vi "Runtime.vi"() -> ()   [LabVIEW 2025]
uses:
  <vilib>/Platform/TimedLoop/XDataNode/timing_clust.ctl
  <vilib>/Platform/TimedLoop/XDataNode/nitl_modes.ctl
  <vilib>/Platform/TimedLoop/XDataNode/wakeup.ctl
  <vilib>/Analysis/5stat.llb/RMS (DBL).vi
  <vilib>/platform/TimedLoop/XDataNode/XDataNode.xnode
  <vilib>/Platform/TimedLoop/XDataNode/XDNodeRunTimeDep.lvlib
  <vilib>/Analysis/NI_AALBase.lvlib
  <vilib>/ptbypt/NI_PtbyPt.lvlib
  <vilib>/Analysis/NI_AALPro.lvlib
panel:
  in  "結束":bool
  out "Velocity":dbl[](graph)
  out "Initial position":i32
  in  "產生路徑":bool
  out "after servo on":u16 format="%.0b"
  out "Initial target velocity":i32
  out "statusword":u16 format="%.0b"
  out "1st Transmit PDO Mapping-Modes of operation display":i8
  in  "Servo on":bool
  in  "1st Receive PDO Mapping-Controlword":u16=128 format="%.0b"
  in  "Fault reset":bool
  in  "STOP":bool
  out "rms error":dbl format="%0.2f"
  out "TCP":errorcluster
  out "Error":string
  out "Done 2":bool caption="TCP Done"
  out "Path":dbl[](graph)
  out "Output":dbl[](graph)
  out "Error":dbl[](graph)
  out "限制上限":bool
  out "Delay":i32
  out "Done":bool caption="Run Done"
  in  "停止":bool
  in  "開始執行":bool
  out "data length":i32
  out "pdl":i32
  out "Total time":i32
  out "Ts":dbl=0.001
  # "資料儲存區"
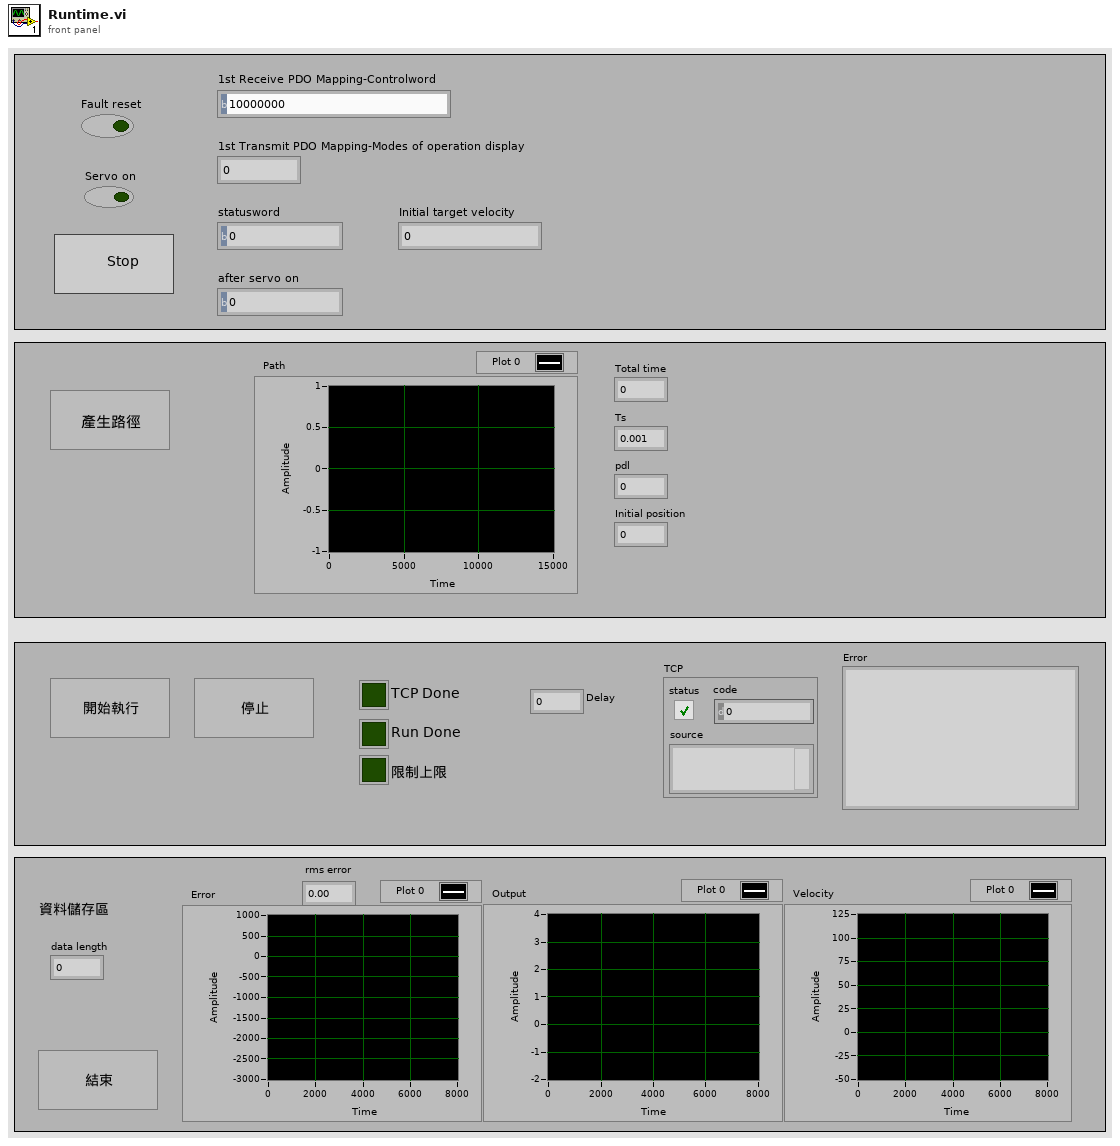
[diagram p1: front panel]
types:
  T1 = typedef "XDNodeRunTimeDep.lvlib/timing_clust.ctl" = cluster{"Expected End [f-1]":u64, "Actual End [f-1]":u64, "Finished Late? [f-1]":bool, "Expected End [i-1]":u64, "Actual End [i-1]":u64, "Finished Late? [i-1]":bool, "Expected Start [i]":u64, "Actual Start [i]":u64, "Expected Start [f]":u64, "Actual Start [f]":u64, "Source Name":string, "Structure Name":string, "Period":i64, "Deadline":i64, "Offset":i64, "Start":i64, "Priority":i32, "Timeout":i32, "Mode":T2, "Wakeup Reason":T3, "Error":errorcluster, "Source Type":string, "Secondary Source Type":string, "Global End Time":u64, "Global Start Time":u64, "Frame Duration":u64, "Iteration Duration":u64, "Assigned CPU":i32, "I/O Scan Engine Mode":u32}
  T2 = typedef "XDNodeRunTimeDep.lvlib/nitl_modes.ctl" = enum32{"No Change", "Process missed periods, maintain original phase", "Discard missed periods, maintain original phase", "Process missed periods, ignore original phase", "Discard missed periods, ignore original phase"}
  T3 = typedef "XDNodeRunTimeDep.lvlib/wakeup.ctl" = enum32{"Normal", "Aborted", "Asynchronous wakeup", "Timing source error", "Timed loop error", "Timeout"}
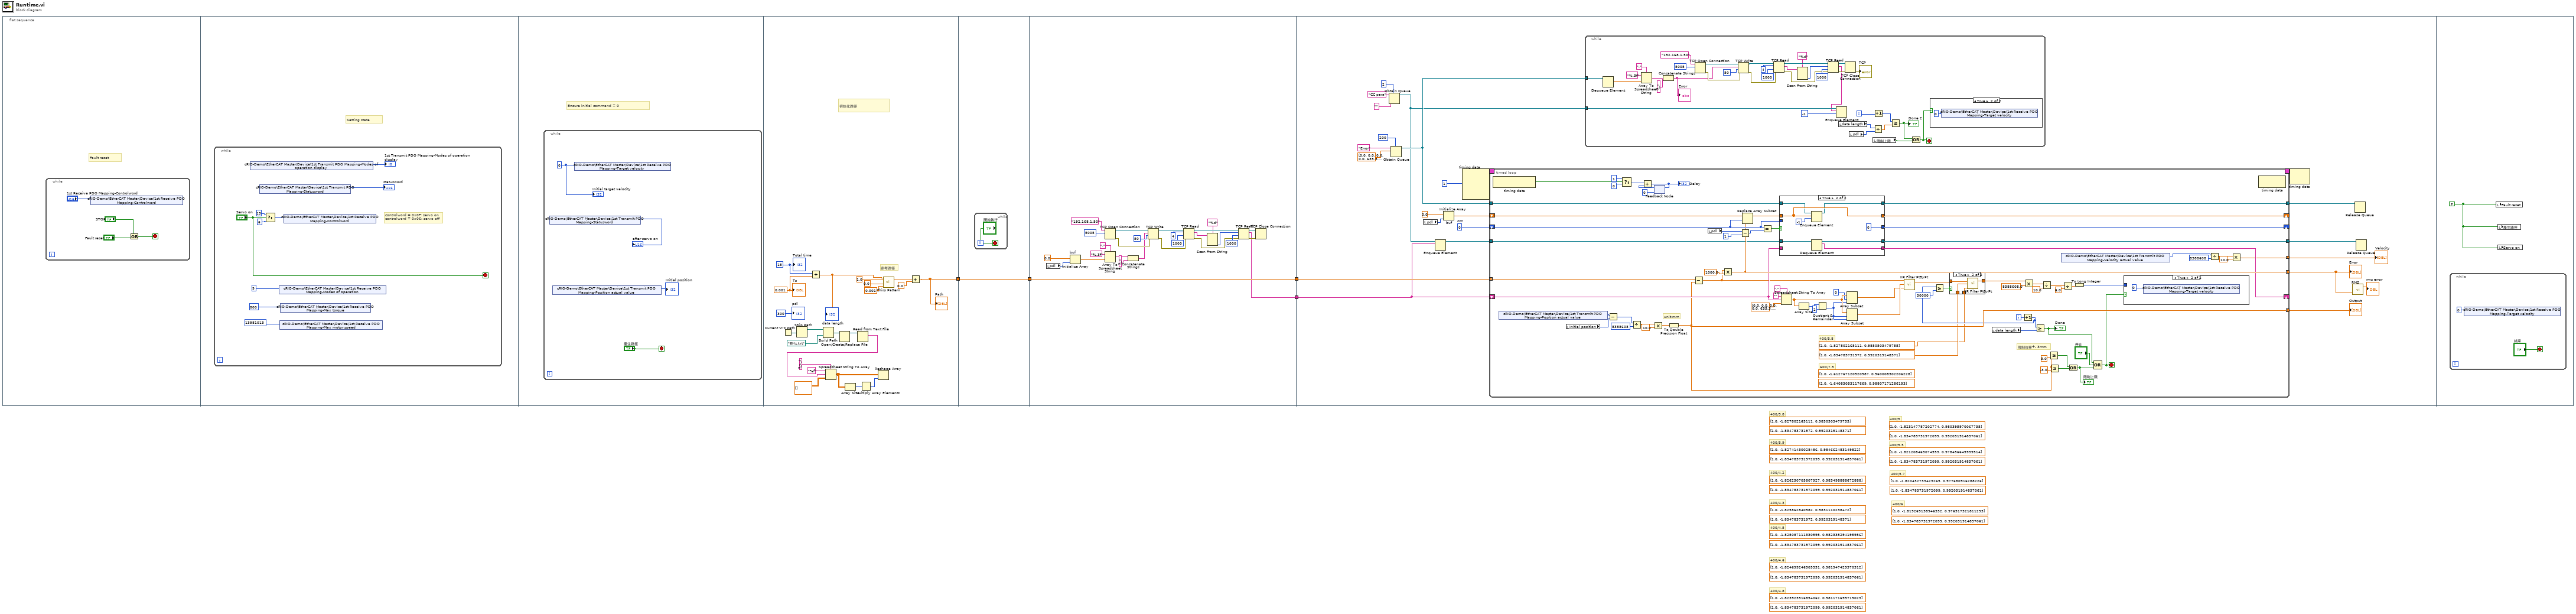
[diagram p0: block diagram]
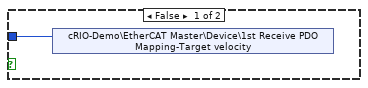
[diagram p4: hidden frame]
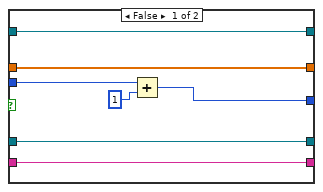
[diagram p5: hidden frame]
diagram:
  (unwired) dbl[] [1.0, -1.834783731972099, 0.992031914837061] ("Numerator")
  (unwired) dbl[] [1.0, -1.820432733423265, 0.977680916288226] ("Numerator")
  (unwired) dbl[] [1.0, -1.834783731972099, 0.992031914837061] ("Numerator")
  (unwired) dbl[] [1.0, -1.819269138946332, 0.976517321811293] ("Numerator")
  (unwired) dbl[] [1.0, -1.834783731972099, 0.992031914837061] ("Numerator")
  (unwired) dbl[] [1.0, -1.821208463074553, 0.978456645939514] ("Numerator")
  (unwired) dbl[] [1.0, -1.834783731972099, 0.992031914837061] ("Numerator")
  (unwired) dbl[] [1.0, -1.823147787202774, 0.980395970067735] ("Numerator")
  (unwired) dbl[] [1.0, -1.834783731972099, 0.992031914837061] ("Numerator")
  (unwired) dbl[] [1.0, -1.823923516854062, 0.981171699719023] ("Numerator")
  (unwired) dbl[] [1.0, -1.834783731972, 0.9920319148371] ("Numerator")
  (unwired) dbl[] [1.0, -1.827802165111, 0.9850503479755] ("Numerator")
  (unwired) dbl[] [1.0, -1.834783731972099, 0.992031914837061] ("Numerator")
  (unwired) dbl[] [1.0, -1.824699246505351, 0.981947429370312] ("Numerator")
  (unwired) dbl[] [1.0, -1.834783731972099, 0.992031914837061] ("Numerator")
  (unwired) dbl[] [1.0, -1.825087111330995, 0.982335294195956] ("Numerator")
  (unwired) dbl[] [1.0, -1.834783731972, 0.9920319148371] ("Numerator")
  (unwired) dbl[] [1.0, -1.825862840982, 0.9831110238472] ("Numerator")
  (unwired) dbl[] [1.0, -1.834783731972099, 0.992031914837061] ("Numerator")
  (unwired) dbl[] [1.0, -1.826250705807927, 0.983498888672888] ("Numerator")
  (unwired) dbl[] [1.0, -1.834783731972099, 0.992031914837061] ("Numerator")
  (unwired) dbl[] [1.0, -1.82741430028486, 0.984662483149822] ("Numerator")
  # "400/5.7"
  # "400/6"
  # "400/5.5"
  # "400/5"
  # "400/4.8"
  # "400/3.8"
  # "400/4.6"
  # "400/4.5"
  # "400/4.3"
  # "400/4.2"
  # "400/3.9"
  n1 = flat-sequence {
    tunnel: [w22] -> w4
    tunnel: [w44] -> w3
    tunnel: w4 -> [w44]
    tunnel: w3 -> [w72]
    tunnel: [w72] -> w2
    tunnel: [w49] -> w1
    tunnel: w2 -> [w93]
    tunnel: w1 -> [w78]
    frame #0 {
      # "Fault reset"
      n2 = while {
        stop <- w6 stop-if-true
        n3 = shared-variable "cRIO-Demo\\EtherCAT Master\\Device\\1st Receive PDO Mapping-Controlword"("1st Receive PDO Mapping-Controlword") -> ()  [unwired: 1 in, 1 out]
        n4 = Or(x="STOP", y="Fault reset") -> (x .or. y?=w6:bool)
      }
    }
    frame #1 {
      # "Setting state"
      n5 = while {
        stop <- "Servo on" stop-if-true
        # "controlword = 0x0F: servo on\ncontrolword = 0x06: servo off"
        n6 = shared-variable "cRIO-Demo\\EtherCAT Master\\Device\\1st Transmit PDO Mapping-Modes of operation display"() -> (→"1st Transmit PDO Mapping-Modes of operation display":i8)  [unwired: 1 in, 1 out]
        n7 = shared-variable "cRIO-Demo\\EtherCAT Master\\Device\\1st Transmit PDO Mapping-Statusword"() -> (→"statusword":u16)  [unwired: 1 in, 1 out]
        n8 = Select(t=u16 15 ("4th Receive PDO Mapping-Controlword"), s="Servo on", f=u16 6 ("4th Receive PDO Mapping-Controlword")) -> (s? t:f=w12:u16)
        n9 = shared-variable "cRIO-Demo\\EtherCAT Master\\Device\\1st Receive PDO Mapping-Modes of operation"(i8 9 ("1st Receive PDO Mapping-Modes of operation")) -> ()  [unwired: 1 in, 1 out]
        n10 = shared-variable "cRIO-Demo\\EtherCAT Master\\Device\\1st Receive PDO Mapping-Max motor speed"(u32 13981013 ("1st Receive PDO Mapping-Max motor speed")) -> ()  [unwired: 1 in, 1 out]
        n11 = shared-variable "cRIO-Demo\\EtherCAT Master\\Device\\1st Receive PDO Mapping-Max torque"(u16 800 ("1st Receive PDO Mapping-Max torque")) -> ()  [unwired: 1 in, 1 out]
        n12 = shared-variable "cRIO-Demo\\EtherCAT Master\\Device\\1st Receive PDO Mapping-Controlword"(w12) -> ()  [unwired: 1 in, 1 out]
      }
    }
    frame #2 {
      # "Ensure initial command = 0"
      n13 = while {
        stop <- "產生路徑" stop-if-true
        w19 = 0 ("1st Receive PDO Mapping-Target position")
        n14 = shared-variable "cRIO-Demo\\EtherCAT Master\\Device\\1st Transmit PDO Mapping-Statusword"() -> (→"after servo on":u16)  [unwired: 1 in, 1 out]
        n15 = shared-variable "cRIO-Demo\\EtherCAT Master\\Device\\1st Transmit PDO Mapping-Position actual value"() -> (→"Initial position":i32)  [unwired: 1 in, 1 out]
        n16 = shared-variable "cRIO-Demo\\EtherCAT Master\\Device\\1st Receive PDO Mapping-Target velocity"(w19) -> ()  [unwired: 1 in, 1 out]
        "Initial target velocity" <- w19
      }
    }
    frame #3 {
      w41 = 15
      w42 = 0.001
      # "參考路徑"
      # "初始化路徑"
      n17 = Current VI's Path() -> (path=w34:path)
      n18 = Strip Path(path=w34) -> (stripped path=w33:path)  [unwired: 1 out]
      n19 = Divide(x=w41, y=w42) -> (x/y=w37:dbl)
      "data length" <- w37
      n20 = Build Path(base path=w33, name or relative path=path "6Hz.txt") -> (appended path=w31:path)
      n21 = Open/Create/Replace File(file path (use dialog)=w31) -> (refnum out=w30:refnum<file>)  [unwired: 5 in, 2 out]
      n22 = Read from Text File(file (use dialog)=w30) -> (text=w27:string)  [unwired: 3 in, 3 out]
      n23 = Spreadsheet String To Array(delimiter (Tab)="\r\n", format string="%f", spreadsheet string=w27, array type (2D Dbl)=dbl[][] []) -> (array=w25:dbl[][])
      n24 = Array Size(array=w25) -> (size(s)=w24:i32[])
      n25 = Multiply Array Elements(1:w24) -> (0:w23:i32)
      n26 = Reshape Array(w25, w23) -> ()  [unwired: 1 out]
      n27 = call <vilib>:"Chirp Pattern.vi"("f2"=0.001, "f1"=0.0, "amplitude"=1.0, "samples"=w37) -> ("Chirp Pattern"=w36:dbl[])  [unwired: 1 out]
      n28 = Add(x=w36, y=0.0) -> (x+y=w22:dbl[])
      "Path" <- w22
      "Ts" <- w42
      "Total time" <- w41
      "pdl" <- 300
    }
    frame #4 {
      n29 = while {
        stop <- "開始執行" stop-if-true
      }
    }
    frame #5 {
      n30 = local read "pdl"() -> (w67:i32)
      n31 = Initialize Array "buf"(0.0 ("element"), w67) -> (w68:dbl[])
      n32 = TCP Open Connection(address="192.168.1.50", remote port or service name=u16 5005) -> (connection ID=w64:refnum<k5>, error out=w53:errorcluster)  [unwired: 3 in]
      n33 = Array To Spreadsheet String(delimiter (Tab)=",", array=w68, 3:"%.3f" ("format string")) -> (spreadsheet string=w48:string)
      n34 = Concatenate Strings(w48, "\n" ("string")) -> (w47:string)
      n35 = TCP Write(connection ID=w64, data in=w47, error in (no error)=w53, 9:50 ("timeout ms (25000)")) -> (connection ID out=w54:refnum<k5>, error out=w52:errorcluster)  [unwired: 1 out]
      n36 = TCP Read(connection ID=w54, bytes to read=4, error in (no error)=w52, 9:1000 ("timeout ms (25000)")) -> (connection ID out=w59:refnum<k5>, data out=w58:string, error out=w55:errorcluster)  [unwired: 1 in]
      n37 = Scan From String(format string="%d", input string=w58) -> (output 1=w57:i32)  [unwired: 3 in, 3 out]
      n38 = TCP Read(connection ID=w59, bytes to read=w57, error in (no error)=w55, 9:1000 ("timeout ms (25000)")) -> (connection ID out=w51:refnum<k5>, data out=w49:string, error out=w50:errorcluster)  [unwired: 1 in]
      n39 = TCP Close Connection(connection ID=w51, error in (no error)=w50) -> ()  [unwired: 1 in, 2 out]
    }
    frame #6 {
      w85 = 0  # cnt
      n40 = Obtain Queue(max queue size (-1, unlimited)=2, name (unnamed)="CC para", element data type="") -> (queue out=w77:refnum<queue>)  [unwired: 2 in, 2 out]
      n41 = Obtain Queue(max queue size (-1, unlimited)=200, name (unnamed)="Error", element data type=dbl[] [0.0, 0.0, 0.0, 0.0, 635.3, -3394.0, 6732.0, -5875.0, 1905.0, 0.0]) -> (queue out=w81:refnum<queue>)  [unwired: 2 in, 2 out]
      n42 = local read "pdl"() -> (w79:i32)
      n43 = Enqueue Element(queue=w77, element=w78) -> (queue out=w76:refnum<queue>)  [unwired: 2 in, 2 out]
      n44 = Initialize Array "buf"(0.0 ("element"), w79) -> (w86:dbl[])
      n45 = node-c288(i64 1 ("Period")) -> (w96:T1)  [unwired: 3 in]
      n46 = timed-loop {
        timing: w96 -> [_]
        timing-out: [_] -> w95
        tunnel: w93 -> [w193] mode=indexing
        tunnel: [w156] -> w92 mode=indexing
        tunnel: [w183] -> w74 mode=indexing
        shift-right: [w187] -> _
        shift-left: w86 -> [w191]
        shift-right: [w186] -> _
        shift-left: w85 -> [w188]
        tunnel: w81 -> [w185]
        tunnel: [w182] -> w83
        tunnel: [w180] -> w82
        tunnel: w76 -> [w181]
        shift-right: [w179] -> _
        shift-left: w78 -> [w171]
        tunnel: [w147] -> w73 mode=indexing
        i -> [w192]
        stop <- w142 stop-if-true
        (unwired) dbl[] [1.0, -1.64083053117669, 0.98807171286193] ("Numerator")
        (unwired) dbl[] [1.0, -1.612767120520987, 0.960008302206228] ("Numerator")
        # "400/3.8"
        # "600/7.5"
        # "unit:mm"
        # "限制位移+- 3mm"
        n47 = node-c288() -> (w195:bool)  [unwired: 1 in]
        n48 = shared-variable "cRIO-Demo\\EtherCAT Master\\Device\\1st Transmit PDO Mapping-Position actual value"() -> (w154:i32)  [unwired: 1 in, 1 out]
        n49 = local read "Initial position"() -> (w153:i32)
        n50 = Subtract(x=w154, y=w153) -> (x-y=w152:i32)
        n51 = Select(t=1, s=w195, f=0) -> (s? t:f=w194:i32)
        n52 = Divide(x=w152, y=8388608) -> (x/y=w155:dbl)
        n53 = Multiply(x=w155, y=10.0) -> (x*y=w163:dbl)
        n54 = feedback #1(0) -> (w197:i32)
        n55 = Add(x=w194, y=w197) -> (x+y=w198:i32)
        "Delay" <- w198
        n56 = feedback-in #1(w198) -> ()
        n57 = To Double Precision Float(number=w163) -> (double precision float=w156:dbl)
        n58 = Subtract(x=w193, y=w156) -> (x-y=w160:dbl)
        n59 = local read "pdl"() -> (w168:i32)
        n60 = Multiply(x=w160, y=1000.0) -> (x*y=w183:dbl)
        n61 = Subtract(x=w168, y=1) -> (x-y=w169:i32)
        n62 = Replace Array Subset(array=w191, new element=w183, index=w188) -> (w189:dbl[])
        n63 = Equal?(x=w188, y=w169) -> (x = y?=w190:bool)
        n64 = case shown="True" w190 {
          tunnel: w189 -> [w218 w226]
          tunnel: w188 -> [w219 _]
          tunnel: [w218 w226] -> w187
          tunnel: [w217 0] -> w186
          tunnel: w185 -> [w216 w225]
          tunnel: [w216 w223] -> w182
          tunnel: w181 -> [w215 w224]
          tunnel: [w215 w222] -> w180
          tunnel: [w214 w221] -> w179
          tunnel: w171 -> [w214 _]
          frame False {
            n65 = Add(x=w219, y=1) -> (x+y=w217:i32)
          }
          frame True {
            n66 = Enqueue Element(queue=w225, element=w226, timeout in ms (-1)=-1) -> (queue out=w223:refnum<queue>)  [unwired: 1 in, 2 out]
            n67 = Dequeue Element(queue=w224) -> (queue out=w222:refnum<queue>, element=w221:string)  [unwired: 2 in, 2 out]
          }
        }
        n68 = Spreadsheet String To Array(delimiter (Tab)=",", format string="", spreadsheet string=w171, array type (2D Dbl)=dbl[] [0.0, 0.0, 0.0, 0.0, 635.3, -3394.0, 6732.0, -5875.0, 1905.0, 0.0]) -> (array=w174:dbl[])
        n69 = Array Size(array=w174) -> (size(s)=w176:i32)
        n70 = Quotient & Remainder(x=w176, y=2) -> (floor(x/y)=w170:i32)  [unwired: 1 out]
        n71 = Array Subset(array=w174, index=0, length=w170) -> (w165:dbl[])
        n72 = Array Subset(array=w174, index=w170, length=w170) -> (w166:dbl[])
        n73 = call <vilib>:"IIR Filter PtByPt.vi"("Forward Coefficients"=w165, "Reverse Coefficients"=w166, "x"=w160) -> ("Filtered x"=w136:dbl)  [unwired: 1 in, 1 out]
        n74 = local read "data length"() -> (w202:i32)
        n75 = Increment(x=w192) -> (x+1=w138:i32)
        n76 = Greater Or Equal?(x=w138, y=30000) -> (x >= y?=w139:bool)
        n77 = case shown="True" w139 {
          tunnel: w136 -> [w207 w211]
          tunnel: [w207 w210] -> w137
          tunnel: dbl[] [1.0, -1.834783731972, 0.9920319148371] ("Numerator") -> [_ w209]
          tunnel: dbl[] [1.0, -1.827802165111, 0.9850503479755] ("Numerator") -> [_ w208]
          frame False {
          }
          frame True {
            n78 = call <vilib>:"IIR Filter PtByPt.vi"("Forward Coefficients"=w208, "Reverse Coefficients"=w209, "x"=w211) -> ("Filtered x"=w210:dbl)  [unwired: 1 in, 1 out]
          }
        }
        n79 = Multiply(x=w137, y=8388608.0) -> (x*y=w158:dbl)
        n80 = Greater Or Equal?(x=w138, y=w202) -> (x >= y?=w201:bool)
        "Done" <- w201
        n81 = Divide(x=w158, y=10.0) -> (x/y=w145:dbl)
        n82 = Greater Or Equal?(x=w156, y=3.0) -> (x >= y?=w204:bool)
        n83 = Less Or Equal?(x=w156, y=-3.0) -> (x <= y?=w203:bool)
        n84 = shared-variable "cRIO-Demo\\EtherCAT Master\\Device\\1st Transmit PDO Mapping-Velocity actual value"() -> (w148:i32)  [unwired: 1 in, 1 out]
        n85 = Divide(x=w145, y=6.0) -> (x/y=w144:dbl)
        n86 = Compound Arithmetic op=OR(w204, w203) -> (w143:bool)
        "限制上限" <- w143
        n87 = To Long Integer(number=w144) -> (32bit integer=w141:i32)
        n88 = Compound Arithmetic op=OR(w201, "停止", w143) -> (w142:bool)
        n89 = case shown="True" w142 {
          tunnel: w141 -> [w212 _]
          frame False {
            n90 = shared-variable "cRIO-Demo\\EtherCAT Master\\Device\\1st Receive PDO Mapping-Target velocity"(w212) -> ()  [unwired: 1 in, 1 out]
          }
          frame True {
            n91 = shared-variable "cRIO-Demo\\EtherCAT Master\\Device\\1st Receive PDO Mapping-Target velocity"(0 ("1st Receive PDO Mapping-Target velocity")) -> ()  [unwired: 1 in, 1 out]
          }
        }
        n92 = Divide(x=w148, y=8388608) -> (x/y=w149:dbl)
        n93 = Multiply(x=w149, y=10.0) -> (x*y=w147:dbl)
        n94 = node-c288() -> ()  [unwired: 1 in, 1 out]
      }
      "Error" <- w74
      "Output" <- w92
      "Velocity" <- w73
      n95 = while {
        tunnel: w81 -> [w130]
        tunnel: w77 -> [w123]
        i -> [w125]
        stop <- w97 stop-if-true
        n96 = Dequeue Element(queue=w130) -> (element=w124:dbl[])  [unwired: 2 in, 3 out]
        n97 = Array To Spreadsheet String(delimiter (Tab)=",", array=w124, 3:"%.3f" ("format string")) -> (spreadsheet string=w102:string)
        n98 = Concatenate Strings(w102, "\n" ("string")) -> (w100:string)
        "Error" <- w100
        n99 = TCP Open Connection(address="192.168.1.50", remote port or service name=u16 5005) -> (connection ID=w119:refnum<k5>, error out=w108:errorcluster)  [unwired: 3 in]
        n100 = TCP Write(connection ID=w119, data in=w100, error in (no error)=w108, 9:50 ("timeout ms (25000)")) -> (connection ID out=w109:refnum<k5>, error out=w107:errorcluster)  [unwired: 1 out]
        n101 = TCP Read(connection ID=w109, bytes to read=4, error in (no error)=w107, 9:1000 ("timeout ms (25000)")) -> (connection ID out=w114:refnum<k5>, data out=w113:string, error out=w110:errorcluster)  [unwired: 1 in]
        n102 = Scan From String(format string="%d", input string=w113) -> (output 1=w112:i32)  [unwired: 3 in, 3 out]
        n103 = TCP Read(connection ID=w114, bytes to read=w112, error in (no error)=w110, 9:1000 ("timeout ms (25000)")) -> (connection ID out=w106:refnum<k5>, data out=w104:string, error out=w105:errorcluster)  [unwired: 1 in]
        n104 = Enqueue Element(queue=w123, element=w104, timeout in ms (-1)=-1) -> ()  [unwired: 1 in, 3 out]
        n105 = local read "data length"() -> (w129:i32)
        n106 = TCP Close Connection(connection ID=w106, error in (no error)=w105) -> (error out=→"TCP":errorcluster)  [unwired: 1 in, 1 out]
        n107 = local read "pdl"() -> (w128:i32)
        n108 = Divide(x=w129, y=w128) -> (x/y=w126:dbl)
        n109 = local read "限制上限"() -> (w98:bool)
        n110 = Increment(x=w125) -> (x+1=w127:i32)
        n111 = Greater Or Equal?(x=w127, y=w126) -> (x >= y?=w99:bool)
        "Done 2" <- w99
        n112 = Compound Arithmetic op=OR(w99, w98) -> (w97:bool)
        n113 = case shown="True" w97 {
          frame False {
          }
          frame True {
            n114 = shared-variable "cRIO-Demo\\EtherCAT Master\\Device\\1st Receive PDO Mapping-Target velocity"(0 ("1st Receive PDO Mapping-Target velocity")) -> ()  [unwired: 1 in, 1 out]
          }
        }
      }
      n115 = node-c288(w95) -> ()  [unwired: 1 out]
      n116 = call-poly <vilib>:"RMS.vi"("X"=w74) -> ("rms value"=→"rms error":dbl)  [unwired: 1 out]
      n117 = Release Queue(queue=w83) -> ()  [unwired: 2 in, 3 out]
      n118 = Release Queue(queue=w82) -> ()  [unwired: 2 in, 3 out]
    }
    frame #7 {
      w236 = FALSE
      n119 = while {
        stop <- "結束" stop-if-true
        n120 = shared-variable "cRIO-Demo\\EtherCAT Master\\Device\\1st Receive PDO Mapping-Target velocity"(0 ("1st Receive PDO Mapping-Target velocity")) -> ()  [unwired: 1 in, 1 out]
      }
      n121 = local write "Fault reset"(w236) -> ()
      n122 = local write "產生路徑"(w236) -> ()
      n123 = local write "Servo on"(w236) -> ()
    }
  }
